vi "CH_LM Config Range.vi"(0 "Meter Index":i32, 1 "Range":dbl=1.0, 3 "Option (Value)":enum16{"MINIMUM", "Value", "MAXIMUM"}(ring)=enum."Value", 5 "error in (no error)":errorcluster, 7 "Timeout / ms (3000)":i32=3000, 8 "Action (query)":bool, 9 "Lock Timeout / ms (1000)":i32=1000) -> (11 "Lock timed out":bool, 14 "Meter Index":i32, 15 "Granted Full Scale Range":dbl, 19 "error out":errorcluster)   [LabVIEW 2012, in "CH_LM.lvlib"]
doc: "This command will set/query the meter measurement range expressed in the units defined under the current measurement mode (Joules or Watts).\n\nThe measurement range is selected by expressing the maximum expected measurement which must be greater than 0.0. The <granted full scale range> value will be the lowest available full scale range that can measure the <maximum expected measurement>. For example, if the list of available ranges is 3mW, 30mW and 300mW and the maximum expected measurement is 10mW, the granted range will be 30mW. The <granted full scale range> will be the top range available if the <maximum expected measurement> exceeds the top range value.\n\n<B>Hint:</B>Using the optional MAX and MIN parameters will result in the maximum or minimum available range, respectively. \n\n<B>Attention:</B> It is possible that the range returned from the query will not be the same as the range selected if auto ranging is active"
uses:
  CH_LM.lvlib
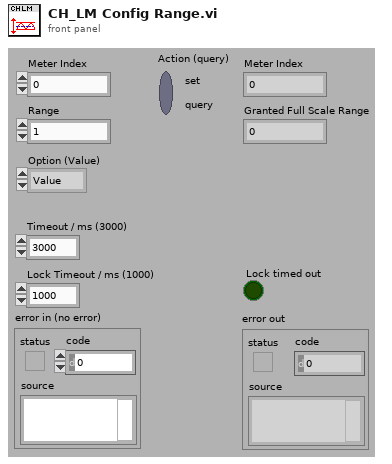
[diagram p1: front panel]
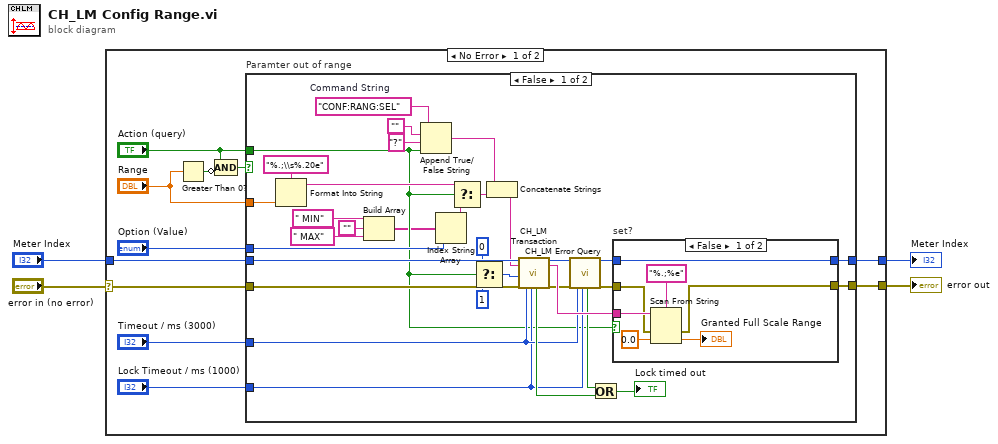
[diagram p0: block diagram]
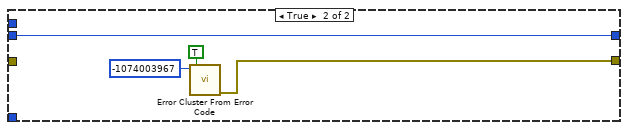
[diagram p3: hidden frame]
diagram:
  n1 = case shown="No Error" "error in (no error)" {
    selector: "error in (no error)" -> [w15 w63]
    tunnel: [w13 w63] -> w4
    tunnel: "Meter Index" -> [w14 w62]
    tunnel: [w11 w62] -> w1
    frame No Error {
      n2 = Greater Than 0?(x="Range") -> (x > 0?=w6:bool)
      n3 = Compound Arithmetic op=AND("Action (query)", invert w6) -> (w7:bool)
      n4 = case "Paramter out of range" shown="False" w7 {
        tunnel: w15 -> [w48 _]
        tunnel: w14 -> [w47 w61]
        tunnel: [w44 w59] -> w13
        tunnel: "Option (Value)" -> [w41 _]
        tunnel: [w35 w61] -> w11
        tunnel: "Timeout / ms (3000)" -> [w27 _]
        tunnel: "Lock Timeout / ms (1000)" -> [w26 _]
        tunnel: "Range" -> [w16 _]
        tunnel: "Action (query)" -> [w25 _]
        frame False {
          w46 = "CONF:RANG:SEL"  # Command String
          n5 = Format Into String(format string="%.;\\s%.20e", w16) -> (resulting string=w40:string)  [unwired: 2 in, 1 out]
          n6 = Build Array(" MIN" ("element"), "", " MAX" ("element")) -> (w20:string[])
          n7 = Append True/False String(1:w25, 2:"?" ("true string"), 3:"", 4:w46) -> (0:w24:string)
          n8 = Index String Array(1:w41, 2:w20) -> (0:w21:string)  [unwired: 1 out]
          n9 = Select(t=w40, s=w25, f=w21) -> (s? t:f=w23:string)
          n10 = Select(t=0, s=w25, f=1 ("NofStrings (-1:all)")) -> (s? t:f=w37:i32)
          n11 = Concatenate Strings(w24, w23) -> (w22:string)
          n12 = call "CH_LM Transaction.vi"("Meter Index"=w47, "Command String"=w22, "NofStrings (-1:all)"=w37, "error in (no error)"=w48, "Timeout / ms (3000)"=w27, "Lock Timeout / ms (1000)"=w26) -> ("Lock timed out"=w29:bool, "Meter Index"=w34:i32, "Response"=w45:string, "error out"=w32:errorcluster)  [unwired: 10 out]
          n13 = call "CH_LM Error Query.vi"("Meter Index"=w34, "error in (no error)"=w32, "Timeout / ms (3000)"=w27, "Lock Timeout / ms (1000)"=w26) -> ("Lock timed out"=w30:bool, "Meter Index"=w33:i32, "error out"=w31:errorcluster)  [unwired: 13 out]
          n14 = Or(x=w30, y=w29) -> (x .or. y?=→"Lock timed out":bool)
          n15 = case "set?" shown="False" w25 {
            tunnel: w45 -> [w55 _]
            tunnel: w31 -> [w54 w57]
            tunnel: [w53 w57] -> w44
            tunnel: w33 -> [w49 w56]
            tunnel: [w49 w56] -> w35
            frame False {
              n16 = Scan From String(format string="%.;%e", input string=w55, error in=w54, default 1=0.0 ("default value 1")) -> (error out=w53:errorcluster, output 1=→"Granted Full Scale Range":dbl)  [unwired: 1 in, 2 out]
            }
            frame True {
            }
          }
        }
        frame True {
          n17 = call <vilib>:"Error Cluster From Error Code.vi"("show call chain? (False)"=TRUE, "error code (0)"=-1074003967) -> ("error out"=w59:errorcluster)  [unwired: 1 in, 6 out]
        }
      }
    }
    frame Error {
    }
  }
  "error out" <- w4
  "Meter Index" <- w1
